vi "Read Deposition file index.vi"(8 "error in (no error)":errorcluster, 11 "BC-Main in":refnum<class "SC-Main.lvclass">) -> (0 "error out":errorcluster, 2 "Deposition file index":i32, 3 "BC-Main out":refnum<class "SC-Main.lvclass">)   [LabVIEW 2013, in "SLMControl.lvlib" / "SC-Main.lvclass"]
uses:
  SC-Main.lvclass
  SC-Main.lvclass/SC-Main.ctl
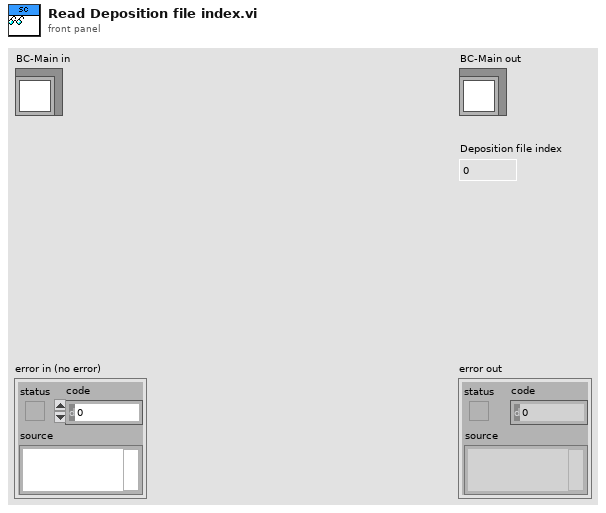
[diagram p1: front panel]
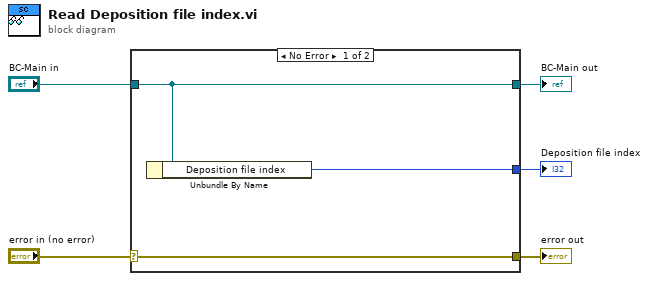
[diagram p0: block diagram]
diagram:
  n1 = case shown="No Error" "error in (no error)" {
    selector: "error in (no error)" -> [w8 w9]
    tunnel: [w8 w9] -> w4
    tunnel: [w7 w10] -> w2
    tunnel: "BC-Main in" -> [w7 w10]
    tunnel: [w6 _] -> w1
    frame No Error {
      n2 = Unbundle By Name(w7) -> ("Deposition file index"=w6:i32)
    }
    frame Error {
    }
  }
  "error out" <- w4
  "BC-Main out" <- w2
  "Deposition file index" <- w1
